vi "Get Chassis IP or Hostname.vi"(0 "session in":refnum<k21>, 5 "chassis":refnum<k21>, 11 "error in (no error)":errorcluster) -> (4 "session out":refnum<k21>, 6 "chassis IP address/hostname":string, 15 "error out":errorcluster)   [LabVIEW 2020, in "SLSC.lvlib"]
doc: "Gets the IP address or hostname of the chassis."
uses:
  <vilib>/SLSC/SLSC.lvlib
  <resource>/objmgr/slsc.rc
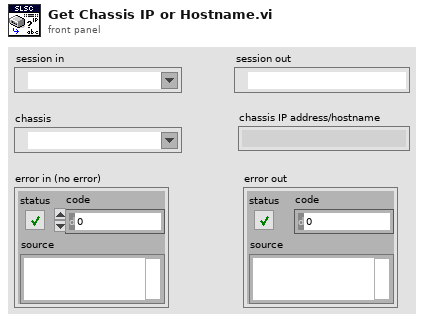
[diagram p1: front panel]
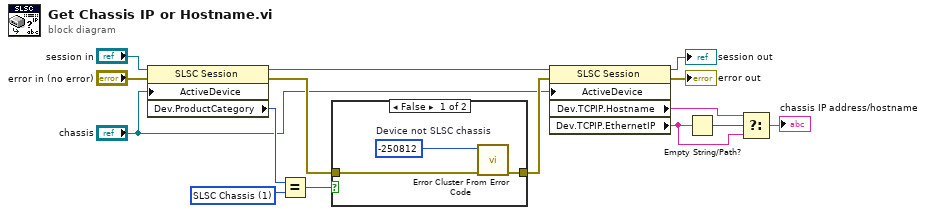
[diagram p0: block diagram]
diagram:
  w8 = 1 items=["Unknown", "SLSC Chassis", "SLSC Module"] ("Dev.ProductCategory")
  n1 = property class="SLSC Session"(reference="session in", error in="error in (no error)", "ActiveDevice"="chassis") -> (reference out=w13:refnum<k21>, error out=w12:errorcluster, "Dev.ProductCategory"=w9:i32)
  n2 = Equal?(x=w9, y=w8) -> (x = y?=w10:bool)
  n3 = case shown="False" w10 {
    tunnel: w12 -> [w18 w19]
    tunnel: [w16 w19] -> w14
    frame False {
      w17 = -250812  # Device not SLSC chassis
      n4 = call <vilib>:"Error Cluster From Error Code.vi"("error in (no error)"=w18, "error code (0)"=w17) -> ("error out"=w16:errorcluster)  [unwired: 7 in]
    }
    frame True {
    }
  }
  n5 = property class="SLSC Session"(reference=w13, error in=w14, "ActiveDevice"="chassis") -> (reference out=→"session out":refnum<k21>, error out=→"error out":errorcluster, "Dev.TCPIP.Hostname"=w2:string, "Dev.TCPIP.EthernetIP"=w15:string)
  n6 = Empty String/Path?(string/path=w15) -> (empty?=w11:bool)
  n7 = Select(t=w2, s=w11, f=w15) -> (s? t:f=→"chassis IP address/hostname":string)
